vi "Check Efficiency.vi"(9 "Rate":dbl, 10 "Gas Mass Flow":dbl, 11 "Eff":dbl) -> (3 "Adjuste Rate":dbl)   [LabVIEW 2023]
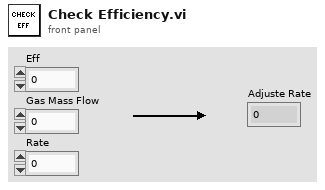
[diagram p1: front panel]
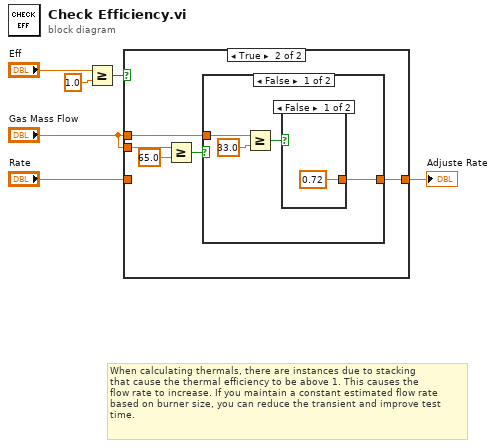
[diagram p0: block diagram]
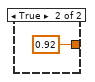
[diagram p3: hidden frame]
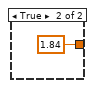
[diagram p4: hidden frame]
diagram:
  # "When calculating thermals, there are instances due to stacking\nthat cause the thermal efficiency to be above 1. This causes the\nflow rate to increase. If you maintain a constant estimated flow rate\nbased on burner size, you can reduce the transient and improve test\ntime."
  n1 = Greater Or Equal?(x="Eff", y=1.0) -> (x >= y?=w3:bool)
  n2 = case shown="True" w3 {
    tunnel: "Gas Mass Flow" -> [_ w12]
    tunnel: "Rate" -> [w7 _]
    tunnel: [w7 w9] -> w5
    tunnel: "Gas Mass Flow" -> [_ w8]
    frame False {
    }
    frame True {
      n3 = Greater Or Equal?(x=w12, y=65.0) -> (x >= y?=w10:bool)
      n4 = case shown="False" w10 {
        tunnel: [w13 1.84 ("y")] -> w9
        tunnel: w8 -> [w15 _]
        frame False {
          n5 = Greater Or Equal?(x=w15, y=33.0) -> (x >= y?=w14:bool)
          n6 = case shown="False" w14 {
            tunnel: [0.72 ("y") 0.92 ("y")] -> w13
            frame False {
            }
            frame True {
            }
          }
        }
        frame True {
        }
      }
    }
  }
  "Adjuste Rate" <- w5
